vi "Read basic params.vi"(0 "device_type in":refnum<class "device_type.lvclass">, 5 "error in (no error)":errorcluster) -> (14 "device_type out":refnum<class "device_type.lvclass">, 15 "buffer size":u32=524288 step=512, 16 "Fs  FPGA":dbl, 17 "SPC":dbl, 18 "center frequency (Hz)":dbl, 19 "error out":errorcluster)   [LabVIEW 2021, in "device_type.lvclass"]
uses:
  device_type.lvclass
  device_type.lvclass/device_type.ctl
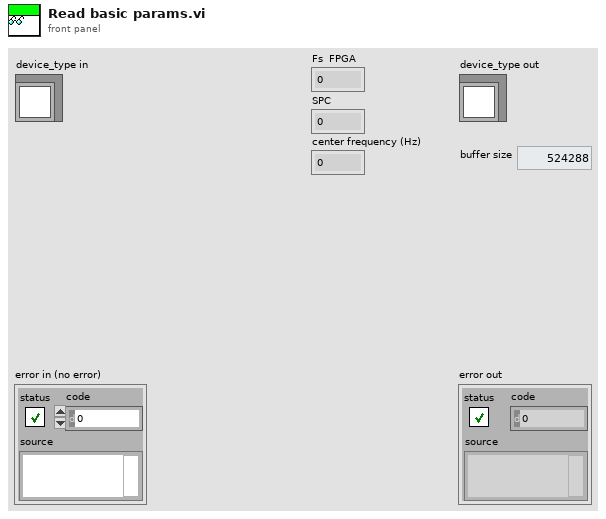
[diagram p1: front panel]
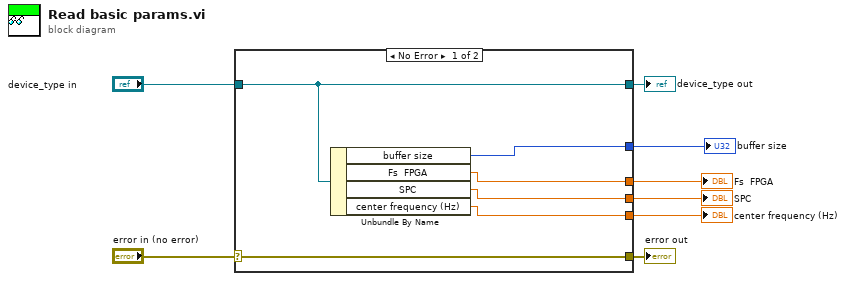
[diagram p0: block diagram]
diagram:
  n1 = case shown="No Error" "error in (no error)" {
    selector: "error in (no error)" -> [w14 w15]
    tunnel: [w14 w15] -> w7
    tunnel: [w13 w16] -> w5
    tunnel: "device_type in" -> [w13 w16]
    tunnel: [w12 _] -> w4
    tunnel: [w11 _] -> w3
    tunnel: [w10 _] -> w2
    tunnel: [w9 _] -> w1
    frame No Error {
      n2 = Unbundle By Name(w13) -> ("buffer size"=w12:u32, "Fs  FPGA"=w9:dbl, "SPC"=w10:dbl, "center frequency (Hz)"=w11:dbl)
    }
    frame Error {
    }
  }
  "error out" <- w7
  "device_type out" <- w5
  "buffer size" <- w4
  "Fs  FPGA" <- w1
  "SPC" <- w2
  "center frequency (Hz)" <- w3
